vi "Write INI.vi"() -> ()   [LabVIEW 2025, in "Scripting Server.lvlib"]
uses:
  Scripting Server.lvlib
  Config Data.ctl
panel:
  in  "Config Data":T1
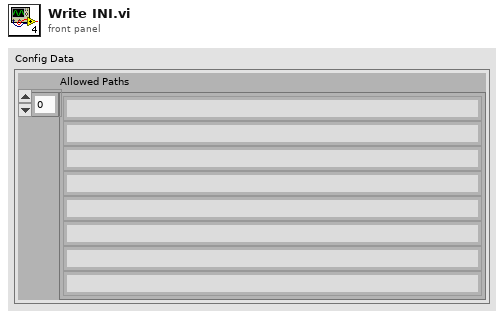
[diagram p1: front panel]
types:
  T1 = typedef "Scripting Server.lvlib/Config Data.ctl" = cluster{"Allowed Paths":string[]}
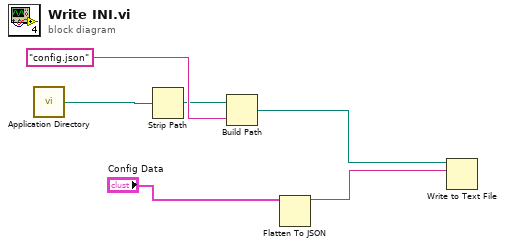
[diagram p0: block diagram]
diagram:
  n1 = call <vilib>:"Application Directory.vi"() -> ("Application Directory"=w4:path)
  n2 = Strip Path(path=w4) -> (stripped path=w5:path)  [unwired: 1 out]
  n3 = Build Path(base path=w5, name or relative path="config.json") -> (appended path=w3:path)
  n4 = Flatten To JSON(anything="Config Data") -> (JSON string=w2:string)  [unwired: 2 in, 1 out]
  n5 = Write to Text File(file (use dialog)=w3, text=w2) -> ()  [unwired: 2 in, 3 out]
